vi "Day 14-Lookup in Polymer Map.vi"(10 "Pair":u8[](array[numeric]), 11 "Polymer Template Map":map{string, string}(c390)) -> (3 "New Entry":u8)   [LabVIEW 2021]
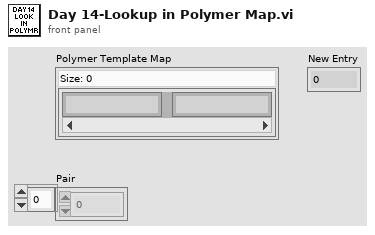
[diagram p1: front panel]
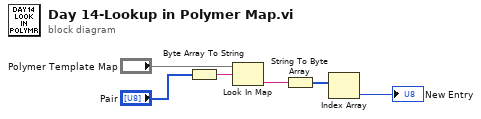
[diagram p0: block diagram]
diagram:
  n1 = Byte Array To String(unsigned byte array="Pair") -> (string=w3:string)
  n2 = Look In Map(map="Polymer Template Map", key=w3) -> (value=w4:string)  [unwired: 1 in, 1 out]
  n3 = String To Byte Array(string=w4) -> (unsigned byte array=w5:u8[])
  n4 = Index Array(array=w5) -> (element=→"New Entry":u8)  [unwired: 1 in]
